vi "AOL Globals Dwell Time updater.vi"(8 "error in":errorcluster, 10 "Disable message (F)":bool) -> (0 "error out":errorcluster)   [LabVIEW 2020]
uses:
  Global Variables/gl_UI Ctrl Refs.vi
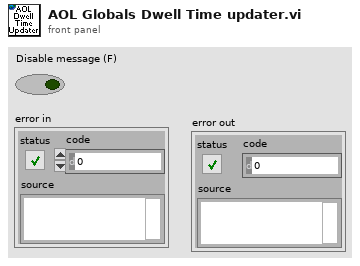
[diagram p1: front panel]
types:
  T1 = typedef "UI ctrl refs cluster.ctl" = cluster{"Top level VI path":path, "Top level VI ref":refnum<vi>, "User menu ref":refnum<k9>, "Sub Panel control":refnum<vi>, "Imaging Param Tab":refnum<vi>, "Occurrence-Start drivers":refnum<k4>, "Occurrence-Speed logging initialised":refnum<k4>, "Occurrence-XYZ stage initialised":refnum<k4>, "Exit button":refnum<vi>, "Status ind":refnum<vi>, "Set as origin":refnum<vi>, "Speed Logging":refnum<vi>, "Time Lapse":refnum<vi>, "Live Imaging":refnum<vi>, "AOL Z Stack":refnum<vi>, "Motor Z Stack":refnum<vi>, "Funct Acq button":refnum<vi>, "Hard Shutter":refnum<vi>, "Virtual Shutter":refnum<vi>, "Laser Power":refnum<vi>, "AOL Mode":refnum<vi>, "Frame Size":refnum<vi>, "Field of View":refnum<vi>, "Dwell Time":refnum<vi>, "Zoom":refnum<vi>, "AOL Z":refnum<vi>, "Objective":refnum<vi>, "Axis":refnum<vi>, "Paths & Names":refnum<vi>, "Experiment folder path (ind.)":refnum<vi>, "Last State (Ind.)":refnum<vi>, "Averages":refnum<vi>, "Angle (degrees)":refnum<vi>, "X centre":refnum<vi>, "Y centre":refnum<vi>, "Plane Mode":refnum<vi>, "# Planes":refnum<vi>, "Z Start":refnum<vi>, "Z Stop":refnum<vi>, "Z Step":refnum<vi>, "PMT 1":refnum<vi>, "PMT 2":refnum<vi>, "Stage XYZ Position":refnum<vi>, "Pockels@Z Start":refnum<vi>, "Pockels@Z Stop":refnum<vi>, "Obtain Z Start":refnum<vi>, "Obtain Z Stop":refnum<vi>, "Live stim.trig.period":refnum<vi>, "Live stim.trig.enable":refnum<vi>, "Movement Correction":refnum<vi>, "Load Reference Image":refnum<vi>, "XY Stage Move":refnum<vi>, "MovCor Cluster":refnum<vi>, "RefDAQParam":refnum<vi>, "Funct. Acq. Pockels Modulation":refnum<vi>, "Ref Laser Power":refnum<vi>, "Enable Video Recording":refnum<vi>, "Video Record-Live Imaging":refnum<vi>, "Video Record-Funct acq":refnum<vi>, "Reference Source":refnum<vi>, "AOL Z-stack Chirps Ready (ind)":refnum<vi>, "Target time between mov.cor. ref triggers (ms)":refnum<vi>, "Funct. Acq. Ref frame save":refnum<vi>, "Tracking button":refnum<vi>, "Show ref plots window":refnum<vi>, "Center freq ind (nm)":refnum<vi>, "Pickup mode (ind)":refnum<vi>, "Logging queue (ind)":refnum<vi>, "Back aperture power (ind.)":refnum<vi>, "Power after objective (ind.)":refnum<vi>, "Switch user":refnum<vi>, "Ls1 Conn. Status":refnum<vi>, "Ls1Tuning Status":refnum<vi>, "Ls1 Faults":refnum<vi>, "Ls1 Connection":refnum<vi>, "Ls1 Mode":refnum<vi>, "Ls1 POWER [mW]":refnum<vi>, "Ls1Shutter":refnum<vi>, "Ls1 Wavelength":refnum<vi>, "Ls1 Note":refnum<vi>, "Ls1 Confirm Wav":refnum<vi>, "Ls1 PreChrp Prism1":refnum<vi>, "Ls1 PreChrp Prism2":refnum<vi>, "Ls1 wav top Ind":refnum<vi>, "Ls1 power top Ind":refnum<vi>, "Ls1 Pump peak Hold":refnum<vi>, "Ls1 Status Ind":refnum<vi>, "Ls1 wav cancel":refnum<vi>, "Experiment Type":refnum<vi>, "Biology Information":refnum<vi>, "Camera recording status":refnum<vi>, "Optimise Obj. Pos.":refnum<vi>}
  T2 = typedef "AOL_Globals.ctl" = cluster{"Imaging Protocol":T3, "Number of POI":u16, "Number of Miniscans":u16, "Number of Trials":u16, "Number of Cycles ":u64, "# Averaged Frames":u16, "Laser power (%)":u8, "Pockels (V)":dbl, "Acquisition Length (sec)":dbl, "Fill time (us)":dbl, "POI Dwell time (us)":dbl, "Miniscan Dwell time per pixel (us)":dbl, "PMT 1":dbl, "PMT 2":dbl, "Back Apperture (mA)":dbl, "Frame Size":T4, "Center Frequency":dbl, "Field of View (um)":dbl, "Field of View (norm)":dbl, "DwellTime (us)":dbl, "Ref Dwell Time (us)":dbl, "Wavelength (nm)":dbl, "Zoom":dbl, "AOL Z":dbl, "AOL Mode":T5, "GridXY":dbl, "GridZ":dbl, "TriggerPeriod (sec)":dbl, "Number of Pixels in Miniscan":u16, "Experiment folder path":path, "X centre":dbl, "Y centre":dbl, "Angle (degrees)":dbl, "Angle Xs (degrees)":dbl, "Angle Ys (degrees)":dbl, "Plane Mode":T6, "Threshold":u16[], "Regenerate Chirps":bool, "Rectangle ROI length (pixels)":u16, "Rectangle ROI height (pixels)":u16, "AOD fill":u16, "StartupDelay":i32, "Samples Wait after Trigger":u16, "Slip Cycle":u32, "Add Cycle":bool, "Functional Mode":T7, "Z Start":dbl, "Z Stop":dbl, "# Planes":i32, "Total Pixels":i32, "Variable Miniscan Pixels":u16[], "Use Variable Length":bool, "Use Variable Resolution":bool, "Laser power (%) at Z Start":u8, "Laser power (%) at Z Stop":u8, "Ref Z Step":i8}
  T3 = typedef "Imaging Protocols enum.ctl" = enum16{"AOL Z-Stack", "Motor Z Stack", "Parameter Sweep", "Functional Acquisition", "Single Plane Acquisition", "Volume Acquisition", "Live Imaging", "Live Plane Imaging", "Live Volume Imaging"}
  T4 = typedef "Frame Size.ctl" = u16
  T5 = typedef "AOL modes.ctl" = enum16{"Raster", "Structural", "Pointing", "Mini Scan", "Alignment"}
  T6 = typedef "Plane Mode.ctl" = u16
  T7 = typedef "Functional Mode.ctl" = enum16{"Point", "Line", "Patch", "Plane", "Volume"}
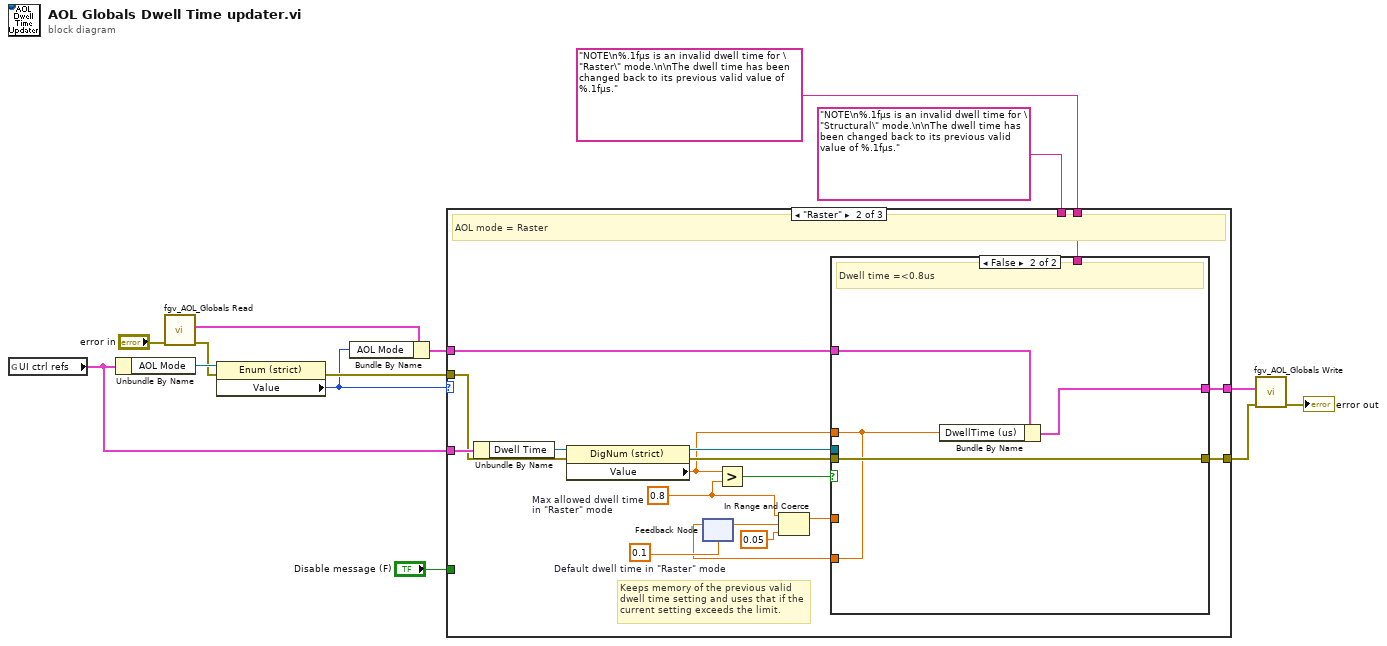
[diagram p0: block diagram]
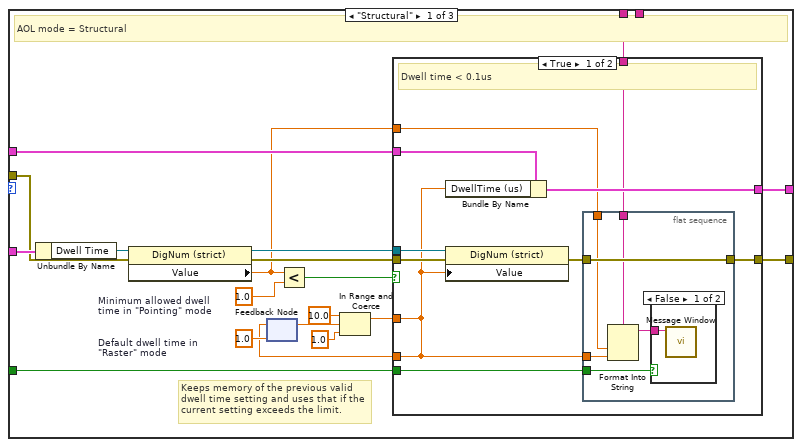
[diagram p2: hidden frame]
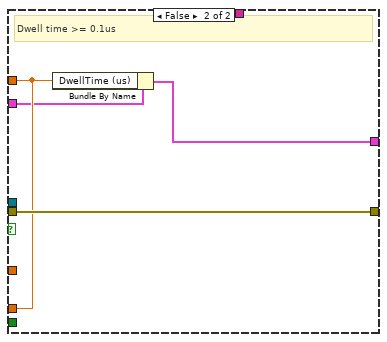
[diagram p4: hidden frame]
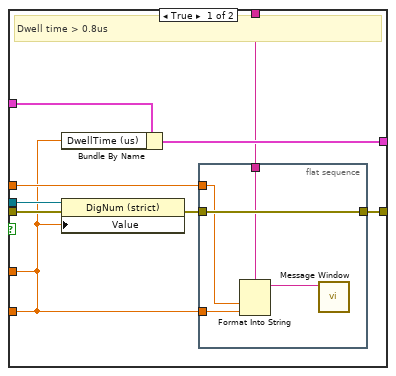
[diagram p5: hidden frame]
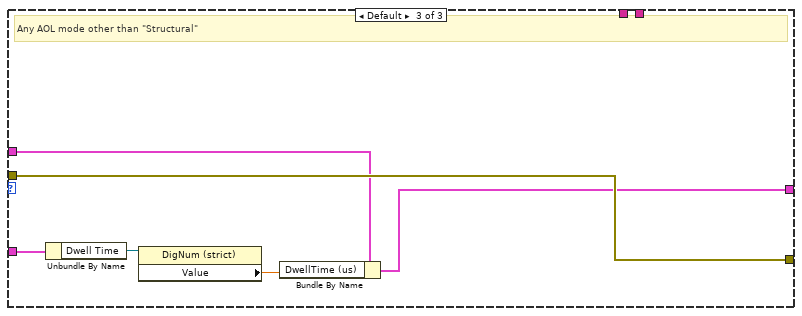
[diagram p6: hidden frame]
diagram:
  n1 = global read "gl_UI Ctrl Refs.vi" "UI ctrl refs"() -> (w12:T1)
  n2 = Unbundle By Name(w12) -> ("AOL Mode"=w14:refnum<vi>)
  n3 = call "fgv_AOL_Globals Read.vi"("error in (no error)"="error in") -> ("error out"=w10:errorcluster, "AOL_Globals"=w5:T2)  [unwired: 8 in, 1 out]
  n4 = property on="Property Node" class="Enum (strict)"(reference=w14, error in=w10) -> (error out=w11:errorcluster, "Value"=w6:T5)  [unwired: 1 out]
  n5 = Bundle By Name(cluster=w5, "AOL Mode"=w6) -> (w4:T2)
  n6 = case shown="\"Raster\"" w6 {
    tunnel: w4 -> [w33 w71 w91]
    tunnel: [w32 w70 w90] -> w13
    tunnel: w12 -> [w30 w68 w93]
    tunnel: w11 -> [w26 w64 w95]
    tunnel: [w25 w63 w95] -> w9
    tunnel: "NOTE\n%.1fµs is an invalid dwell time for \"Structural\" mode.\n\nThe dwell time has been changed back to its previous valid value of %.1fµs." ("Message string") -> [w18 _ _]
    tunnel: "NOTE\n%.1fµs is an invalid dwell time for \"Raster\" mode.\n\nThe dwell time has been changed back to its previous valid value of %.1fµs." ("Message string") -> [_ w58 _]
    tunnel: "Disable message (F)" -> [w15 _ _]
    frame "Structural" {
      w24 = 1.0  # Default dwell time in "Raster" mode
      w20 = 1.0  # Minimum allowed dwell time in "Pointing" mode
      # "Keeps memory of the previous valid dwell time setting and uses that if the current setting exceeds the limit."
      # "AOL mode = Structural"
      n7 = Unbundle By Name(w30) -> ("Dwell Time"=w31:refnum<vi>)
      n8 = property on="Property Node" class="DigNum (strict)"(reference=w31, error in=w26) -> (reference out=w28:refnum<vi>, error out=w27:errorcluster, "Value"=w17:dbl)
      n9 = feedback #1(w24) -> (w23:dbl)
      n10 = Less?(x=w17, y=w20) -> (x < y?=w29:bool)
      n11 = In Range and Coerce(upper limit=10.0, x=w23, lower limit=1.0) -> (coerced(x)=w19:dbl)  [unwired: 1 out]
      n12 = case shown="True" w29 {
        tunnel: w33 -> [w43 w52]
        tunnel: [w42 w51] -> w32
        tunnel: w28 -> [w41 _]
        tunnel: w19 -> [w35 _]
        tunnel: w27 -> [w40 w54]
        tunnel: [w38 w54] -> w25
        tunnel: w18 -> [w37 _]
        tunnel: w17 -> [w36 w53]
        tunnel: [w35 w53] -> w16
        tunnel: w15 -> [w34 _]
        frame True {
          # "Dwell time < 0.1us"
          n13 = Bundle By Name(cluster=w43, "DwellTime (us)"=w35) -> (w42:T2)
          n14 = property on="Property Node" class="DigNum (strict)"(reference=w41, error in=w40, "Value"=w35) -> (error out=w39:errorcluster)  [unwired: 1 out]
          n15 = flat-sequence {
            tunnel: w39 -> [w49]
            tunnel: [w49] -> w38
            tunnel: w35 -> [w46]
            tunnel: w37 -> [w47]
            tunnel: w36 -> [w45]
            tunnel: w34 -> [w44]
            frame #0 {
              n16 = Format Into String(format string=w47, w45, w46) -> (resulting string=w48:string)  [unwired: 2 in, 1 out]
              n17 = case shown="False" w44 {
                tunnel: w48 -> [w50 _]
                frame False {
                  n18 = call "Message Window.vi"("Message string"=w50) -> ()  [unwired: 10 in, 1 out]
                }
                frame True {
                }
              }
            }
          }
        }
        frame False {
          # "Dwell time >= 0.1us"
          n19 = Bundle By Name(cluster=w52, "DwellTime (us)"=w53) -> (w51:T2)
        }
      }
      n20 = feedback-in #1(w16) -> ()
    }
    frame "Raster" {
      w62 = 0.1  # Default dwell time in "Raster" mode
      w59 = 0.8  # Max allowed dwell time in "Raster" mode
      # "Keeps memory of the previous valid dwell time setting and uses that if the current setting exceeds the limit."
      # "AOL mode = Raster"
      n21 = Unbundle By Name(w68) -> ("Dwell Time"=w69:refnum<vi>)
      n22 = property on="Property Node" class="DigNum (strict)"(reference=w69, error in=w64) -> (reference out=w66:refnum<vi>, error out=w65:errorcluster, "Value"=w57:dbl)
      n23 = feedback #2(w62) -> (w61:dbl)
      n24 = Greater?(x=w57, y=w59) -> (0:w67:bool)
      n25 = In Range and Coerce(upper limit=w59, x=w61, lower limit=0.05) -> (coerced(x)=w56:dbl)  [unwired: 1 out]
      n26 = case shown="False" w67 {
        tunnel: w71 -> [w80 w87]
        tunnel: [w79 w86] -> w70
        tunnel: w66 -> [w78 _]
        tunnel: w56 -> [w72 _]
        tunnel: w65 -> [w77 w89]
        tunnel: [w75 w89] -> w63
        tunnel: w58 -> [w74 _]
        tunnel: w57 -> [w73 w88]
        tunnel: [w72 w88] -> w55
        frame True {
          # "Dwell time > 0.8us"
          n27 = Bundle By Name(cluster=w80, "DwellTime (us)"=w72) -> (w79:T2)
          n28 = property on="Property Node" class="DigNum (strict)"(reference=w78, error in=w77, "Value"=w72) -> (error out=w76:errorcluster)  [unwired: 1 out]
          n29 = flat-sequence {
            tunnel: w76 -> [w85]
            tunnel: [w85] -> w75
            tunnel: w72 -> [w82]
            tunnel: w74 -> [w83]
            tunnel: w73 -> [w81]
            frame #0 {
              n30 = Format Into String(format string=w83, w81, w82) -> (resulting string=w84:string)  [unwired: 2 in, 1 out]
              n31 = call "Message Window.vi"("Message string"=w84) -> ()  [unwired: 10 in, 1 out]
            }
          }
        }
        frame False {
          # "Dwell time =<0.8us"
          n32 = Bundle By Name(cluster=w87, "DwellTime (us)"=w88) -> (w86:T2)
        }
      }
      n33 = feedback-in #2(w55) -> ()
    }
    frame Default {
      # "Any AOL mode other than \"Structural\""
      n34 = Unbundle By Name(w93) -> ("Dwell Time"=w94:refnum<vi>)
      n35 = property on="Property Node" class="DigNum (strict)"(reference=w94) -> ("Value"=w92:dbl)  [unwired: 1 in, 2 out]
      n36 = Bundle By Name(cluster=w91, "DwellTime (us)"=w92) -> (w90:T2)
    }
  }
  n37 = call "fgv_AOL_Globals Write.vi"("error in (no error)"=w9, "AOL_Globals"=w13) -> ("error out"=→"error out":errorcluster)  [unwired: 9 in]
